vi "Qualification 1.vi"() -> ()   [LabVIEW 2014]
uses:
  <vilib>/myRIO/Common/Instrument Driver Framework/myRIO v1.0/DIO/typedefs/DIO Channels Enum.ctl
  <vilib>/myRIO/Common/Instrument Driver Framework/myRIO v1.0/DIO/typedefs/DIO Channels List.ctl
  <vilib>/myRIO/Common/Instrument Driver Framework/Utilities/typedefs/Generic FPGA Reference.ctl
  <vilib>/myRIO/Common/Instrument Driver Framework/Utilities/typedefs/myRIO v1.0 Reference.ctl
  <vilib>/myRIO/Common/Instrument Driver Framework/Utilities/typedefs/Hardware Version Enum.ctl
  <vilib>/myRIO/Common/Instrument Driver Framework/Utilities/typedefs/myRIO Generic Hardware Reference.ctl
  <vilib>/myRIO/Instrument Drivers/Onboard IO/DIO/typedefs/DIO Reference.ctl
  <vilib>/myRIO/Instrument Drivers/Onboard IO/DIO/DIO.lvlib
  <vilib>/myRIO/Instrument Drivers/Onboard IO/DIO/vis/Write.vi
  <vilib>/userdefined/High Color/nirio_resource_hc.ctl
  <vilib>/myRIO/Common/Instrument Driver Framework/myRIO v1.0/DIO/vis/myRIO v1.1 Open DIO.vi
  <vilib>/myRIO/Instrument Drivers/Onboard IO/DIO/vis/myRIO DIO Open.xnode
  <vilib>/myRIO/Common/Instrument Driver Framework/Utilities/vis/Is FPGA Ref Available.vi
  <vilib>/myRIO/Express VI/Onboard IO/DO/DO Express VI.xnode
  <vilib>/myRIO/Instrument Drivers/Onboard IO/DIO/vis/Read.vi
  <vilib>/myRIO/Express VI/Onboard IO/DI/DI Express VI.xnode
  <vilib>/functionblocks/FB Core/FB Core.xnode
  <vilib>/myRIO/Express VI/Onboard Devices/LED/LED Express VI.xnode
  <vilib>/myRIO/Instrument Drivers/Utilities/Utilities.lvlib
  <vilib>/functionblocks/Edge Detection/One Shot Falling With Input/One Shot Falling With Input.vi
  <vilib>/functionblocks/NI_FunctionBlock Libraries.lvlib
panel:
  in  "stop 2":bool
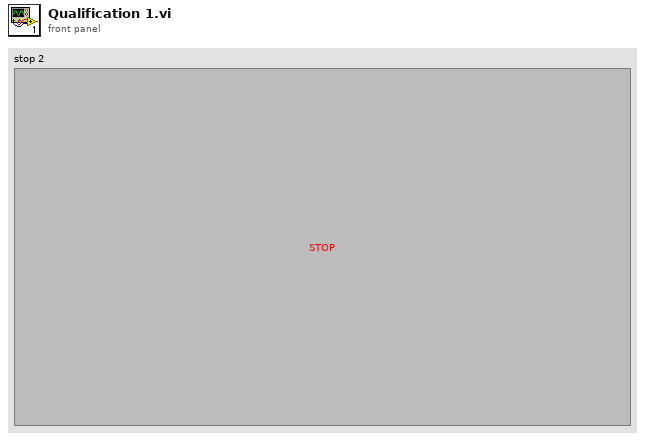
[diagram p1: front panel]
types:
  T1 = typedef "DIO.lvlib/DIO Reference.ctl" = cluster{"myRIO Reference":T2, "DIO Channels List":T6}
  T2 = typedef "myRIO Generic Hardware Reference.ctl" = cluster{"myRIO Model":T3, "myRIO Hardware Reference":T4}
  T3 = typedef "Hardware Version Enum.ctl" = enum16{"Unknown", "myRIO-1900", "myRIO-1950"}
  T4 = typedef "myRIO v1.0 Reference.ctl" = cluster{"Generic FPGA Reference":T5, "Allow multiple opens":bool}
  T5 = typedef "Generic FPGA Reference.ctl" = refnum<k20>
  T6 = typedef "DIO Channels List.ctl" = T7[]
  T7 = typedef "DIO Channels Enum.ctl" = enum16{"Not Connected", "C/DIO0", "C/DIO1", "C/DIO2", "C/DIO3", "C/DIO4", "C/DIO5", "C/DIO6", "C/DIO7", "A/DIO0", "A/DIO1", "A/DIO2", "A/DIO3", "A/DIO4", "A/DIO5", "A/DIO6", "A/DIO7", "A/DIO8", "A/DIO9", "A/DIO10", "A/DIO11", "A/DIO12", "A/DIO13", "A/DIO14", "A/DIO15", "B/DIO0", "B/DIO1", "B/DIO2", "B/DIO3", "B/DIO4", "B/DIO5", "B/DIO6", "B/DIO7", "B/DIO8", "B/DIO9", "B/DIO10", "B/DIO11", "B/DIO12", "B/DIO13", "B/DIO14", "B/DIO15", "LED0", "LED1", "LED2", "LED3", "Button0"}
  T8 = typedef "nirio_resource_hc.ctl" = tag
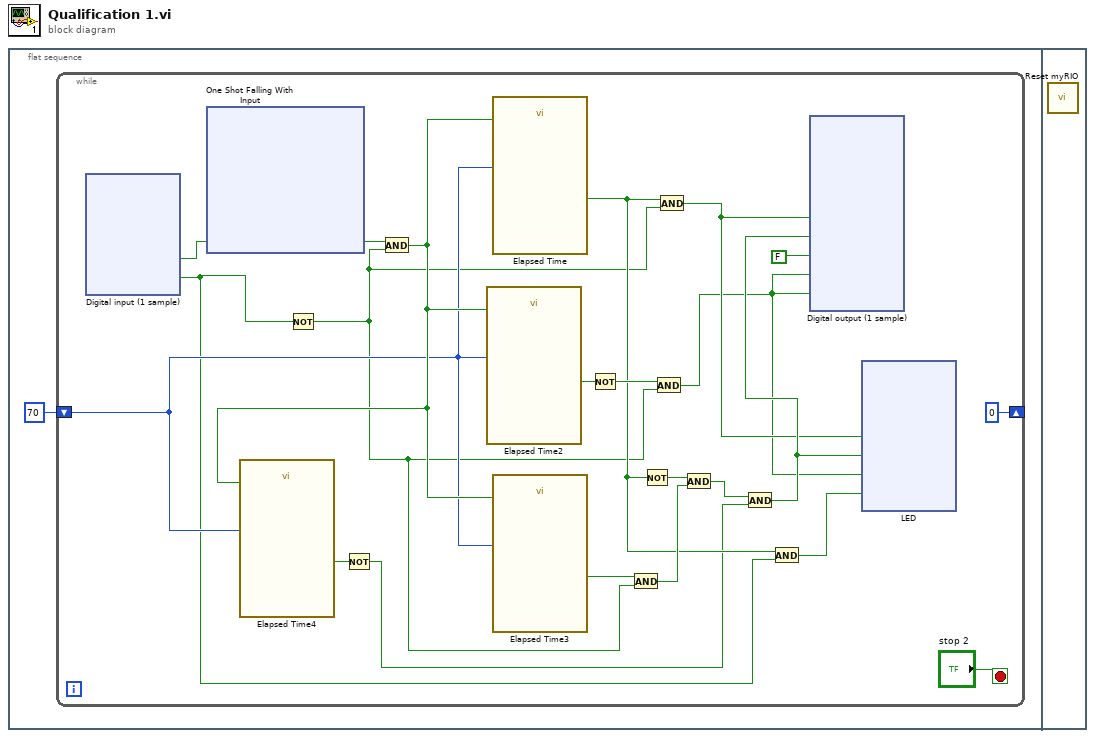
[diagram p0: block diagram]
diagram:
  n1 = flat-sequence {
    frame #0 {
      n2 = while {
        shift-right: [0] -> _
        shift-left: 70 -> [w12]
        stop <- "stop 2" stop-if-true
        n3 = xnode "Digital input (1 sample)"() -> ("B/DIO2 (Pin 15)"=w15:bool, "B/DIO5 (Pin 21)"=w4:bool)  [unwired: 1 in, 1 out]
        n4 = xnode "One Shot Falling With Input"("input"=w15) -> ("output"=w13:bool)  [unwired: 1 in, 1 out]
        n5 = Not(x=w4) -> (.not. x?=w2:bool)
        n6 = And(x=w13, y=w2) -> (x .and. y?=w14:bool)
        n7 = call "Elapsed Time4"("Reset"=w14, "Set Start Time (s)"=w12) -> ("Time has Elapsed"=w19:bool)  [unwired: 10 in, 7 out]
        n8 = Not(x=w19) -> (.not. x?=w3:bool)
        n9 = call "Elapsed Time2"("Reset"=w14, "Set Start Time (s)"=w12) -> ("Time has Elapsed"=w21:bool)  [unwired: 10 in, 7 out]
        n10 = call "Elapsed Time"("Reset"=w14, "Set Start Time (s)"=w12) -> ("Time has Elapsed"=w5:bool)  [unwired: 10 in, 7 out]
        n11 = call "Elapsed Time3"("Reset"=w14, "Set Start Time (s)"=w12) -> ("Time has Elapsed"=w9:bool)  [unwired: 10 in, 7 out]
        n12 = Not(x=w21) -> (.not. x?=w8:bool)
        n13 = And(x=w9, y=w2) -> (x .and. y?=w10:bool)
        n14 = Not(x=w5) -> (.not. x?=w20:bool)
        n15 = And(x=w8, y=w2) -> (x .and. y?=w7:bool)
        n16 = And(x=w5, y=w2) -> (x .and. y?=w11:bool)
        n17 = And(x=w20, y=w10) -> (x .and. y?=w18:bool)
        n18 = And(x=w18, y=w3) -> (x .and. y?=w17:bool)
        n19 = And(x=w5, y=w4) -> (x .and. y?=w6:bool)
        n20 = xnode "Digital output (1 sample)"("A/DIO6 (Pin 23)"=w11, "A/DIO7 (Pin 25)"=w17, "A/DIO14 (Pin 32)"=FALSE ("A/DIO7 (Pin 25)"), "A/DIO15 (Pin 34)"=w7, "A/DIO0 (Pin 11)"=w7) -> ()  [unwired: 1 in, 1 out]
        n21 = xnode "LED"("LED0"=w11, "LED1"=w17, "LED2"=w7, "LED3"=w6) -> ()  [unwired: 1 in, 1 out]
      }
    }
    frame #1 {
      n22 = call <vilib>:"Reset myRIO.vi"() -> ()  [unwired: 11 in, 1 out]
    }
  }
